vi "PathPlanner_Path_RePlan_Worker4.vi"(0 "JoinAnchor":T1 {"Y" format="%14.3f"; "X" format="%14.3f"}, 4 "StartingPoseTranslation":T1 {"Y" format="%14.3f"; "X" format="%14.3f"}, 5 "in PathPlannerPath":T2 {"AllPoints"."HolonomicRotation"."SIN" format="%13.4f"; "AllPoints"."HolonomicRotation"."COS" format="%13.4f"; "AllPoints"."HolonomicRotation"."VALUE" format="%13.4f"; "AllPoints"."Position"."Y" format="%14.3f"; "AllPoints"."Position"."X" format="%14.3f"; "GoalEndState"."Rotation"."SIN" format="%13.4f"; "GoalEndState"."Rotation"."COS" format="%13.4f"; "GoalEndState"."Rotation"."VALUE" format="%13.4f"; "RotationTargets"."target"."SIN" format="%13.4f"; "RotationTargets"."target"."COS" format="%13.4f"; "RotationTargets"."target"."VALUE" format="%13.4f"; "PreviewStartingRotation"."SIN" format="%13.4f"; "PreviewStartingRotation"."COS" format="%13.4f"; "PreviewStartingRotation"."VALUE" format="%13.4f"; "BezierPoints"."Y" format="%14.3f"; "BezierPoints"."X" format="%14.3f"}, 6 "robotNextCtrl":T1 {"Y" format="%14.3f"; "X" format="%14.3f"}, 7 "NumPtsMinusOne":i32, 9 "robotNextCtrl_NULL":bool, 10 "JoinPrevCtrl":T1 {"Y" format="%14.3f"; "X" format="%14.3f"}) -> (2 "Error":bool, 3 "Replanned Path":T2 {"AllPoints"."HolonomicRotation"."SIN" format="%13.4f"; "AllPoints"."HolonomicRotation"."COS" format="%13.4f"; "AllPoints"."HolonomicRotation"."VALUE" format="%13.4f"; "AllPoints"."Position"."Y" format="%14.3f"; "AllPoints"."Position"."X" format="%14.3f"; "GoalEndState"."Rotation"."SIN" format="%13.4f"; "GoalEndState"."Rotation"."COS" format="%13.4f"; "GoalEndState"."Rotation"."VALUE" format="%13.4f"; "RotationTargets"."target"."SIN" format="%13.4f"; "RotationTargets"."target"."COS" format="%13.4f"; "RotationTargets"."target"."VALUE" format="%13.4f"; "PreviewStartingRotation"."SIN" format="%13.4f"; "PreviewStartingRotation"."COS" format="%13.4f"; "PreviewStartingRotation"."VALUE" format="%13.4f"; "BezierPoints"."Y" format="%14.3f"; "BezierPoints"."X" format="%14.3f"})   [LabVIEW 2019, in "PathPlanner24.lvlib"]
doc: "Replan path worker 4\n\nInternal routine. Not for end user use."
uses:
  PathPlanner24.lvlib
  <vilib>/Rock Robotics/WPI/ThirdParty/JAS_Junk/TrajLib/Trajectory_Library.lvlib
  <vilib>/Rock Robotics/WPI/ThirdParty/JAS_Junk/TrajLib/TypeDef/ROTATION2D.ctl
  TypeDef/PathPlannerRotationTarget.ctl
  TypeDef/PathPlannerPathConstraints.ctl
  TypeDef/PathPlannerConstraintsZone.ctl
  ENum/PathPlanner_CommandUtilType_ENUM.ctl
  TypeDef/PathPlannerCommandUtil.ctl
  TypeDef/PathPlannerEventMarker.ctl
  <vilib>/Rock Robotics/WPI/ThirdParty/JAS_Junk/TrajLib/TypeDef/TRANSLATION2D.ctl
  TypeDef/PathPlannerGoalEndState.ctl
  TypeDef/PathPlannerPathPoint.ctl
  TypeDef/PathPlannerPath.ctl
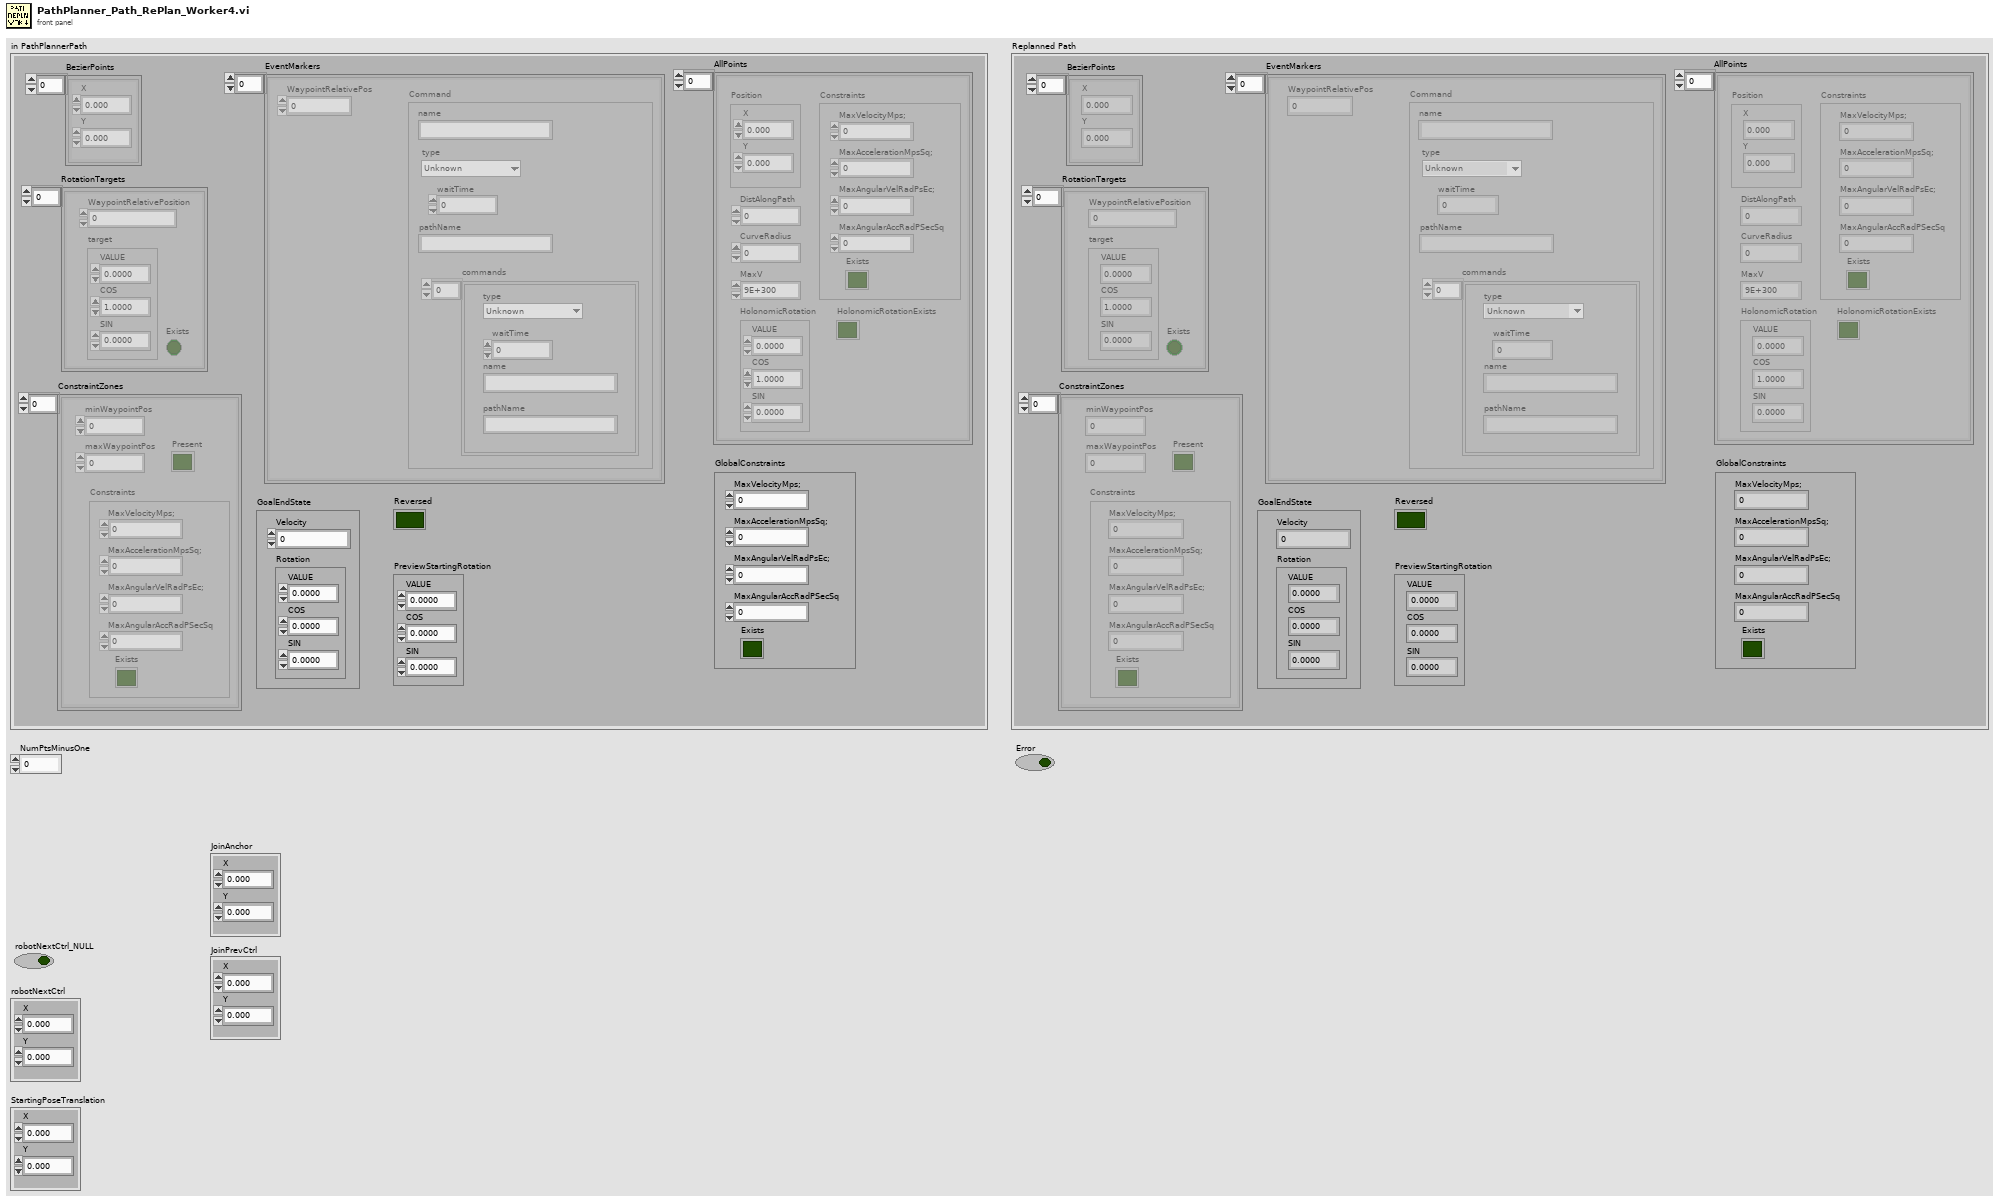
[diagram p1: front panel]
types:
  T1 = typedef "Trajectory_Library.lvlib/TRANSLATION2D.ctl" = cluster{"X":dbl, "Y":dbl}
  T2 = typedef "PathPlanner24.lvlib/PathPlannerPath.ctl" = cluster{"BezierPoints":T1[], "PreviewStartingRotation":T3, "Reversed":bool, "RotationTargets":T4[], "ConstraintZones":T5[], "EventMarkers":T7[], "GlobalConstraints":T6, "GoalEndState":T10, "AllPoints":T11[]}
  T3 = typedef "Trajectory_Library.lvlib/ROTATION2D.ctl" = cluster{"VALUE":dbl, "COS":dbl, "SIN":dbl}
  T4 = typedef "PathPlanner24.lvlib/PathPlannerRotationTarget.ctl" = cluster{"target":T3, "WaypointRelativePosition":dbl, "Exists":bool}
  T5 = typedef "PathPlanner24.lvlib/PathPlannerConstraintsZone.ctl" = cluster{"minWaypointPos":dbl, "maxWaypointPos":dbl, "Constraints":T6, "Present":bool}
  T6 = typedef "PathPlanner24.lvlib/PathPlannerPathConstraints.ctl" = cluster{"MaxVelocityMps;":dbl, "MaxAccelerationMpsSq;":dbl, "MaxAngularVelRadPsEc;":dbl, "MaxAngularAccRadPSecSq":dbl, "Exists":bool}
  T7 = typedef "PathPlanner24.lvlib/PathPlannerEventMarker.ctl" = cluster{"WaypointRelativePos":dbl, "Command":T8}
  T8 = typedef "PathPlanner24.lvlib/PathPlannerCommandUtil.ctl" = cluster{"waitTime":dbl, "name":string, "pathName":string, "commands":cluster{"type":T9, "waitTime":dbl, "name":string, "pathName":string}[], "type":T9}
  T9 = typedef "PathPlanner24.lvlib/PathPlanner_CommandUtilType_ENUM.ctl" = enum16{"Unknown", "Wait", "Named", "Path", "Sequential", "Parallel", "Race", "Deadline"}
  T10 = typedef "PathPlanner24.lvlib/PathPlannerGoalEndState.ctl" = cluster{"Velocity":dbl, "Rotation":T3}
  T11 = typedef "PathPlanner24.lvlib/PathPlannerPathPoint.ctl" = cluster{"Position":T1, "HolonomicRotation":T3, "DistAlongPath":dbl, "CurveRadius":dbl, "MaxV":dbl, "Constraints":T6, "HolonomicRotationExists":bool}
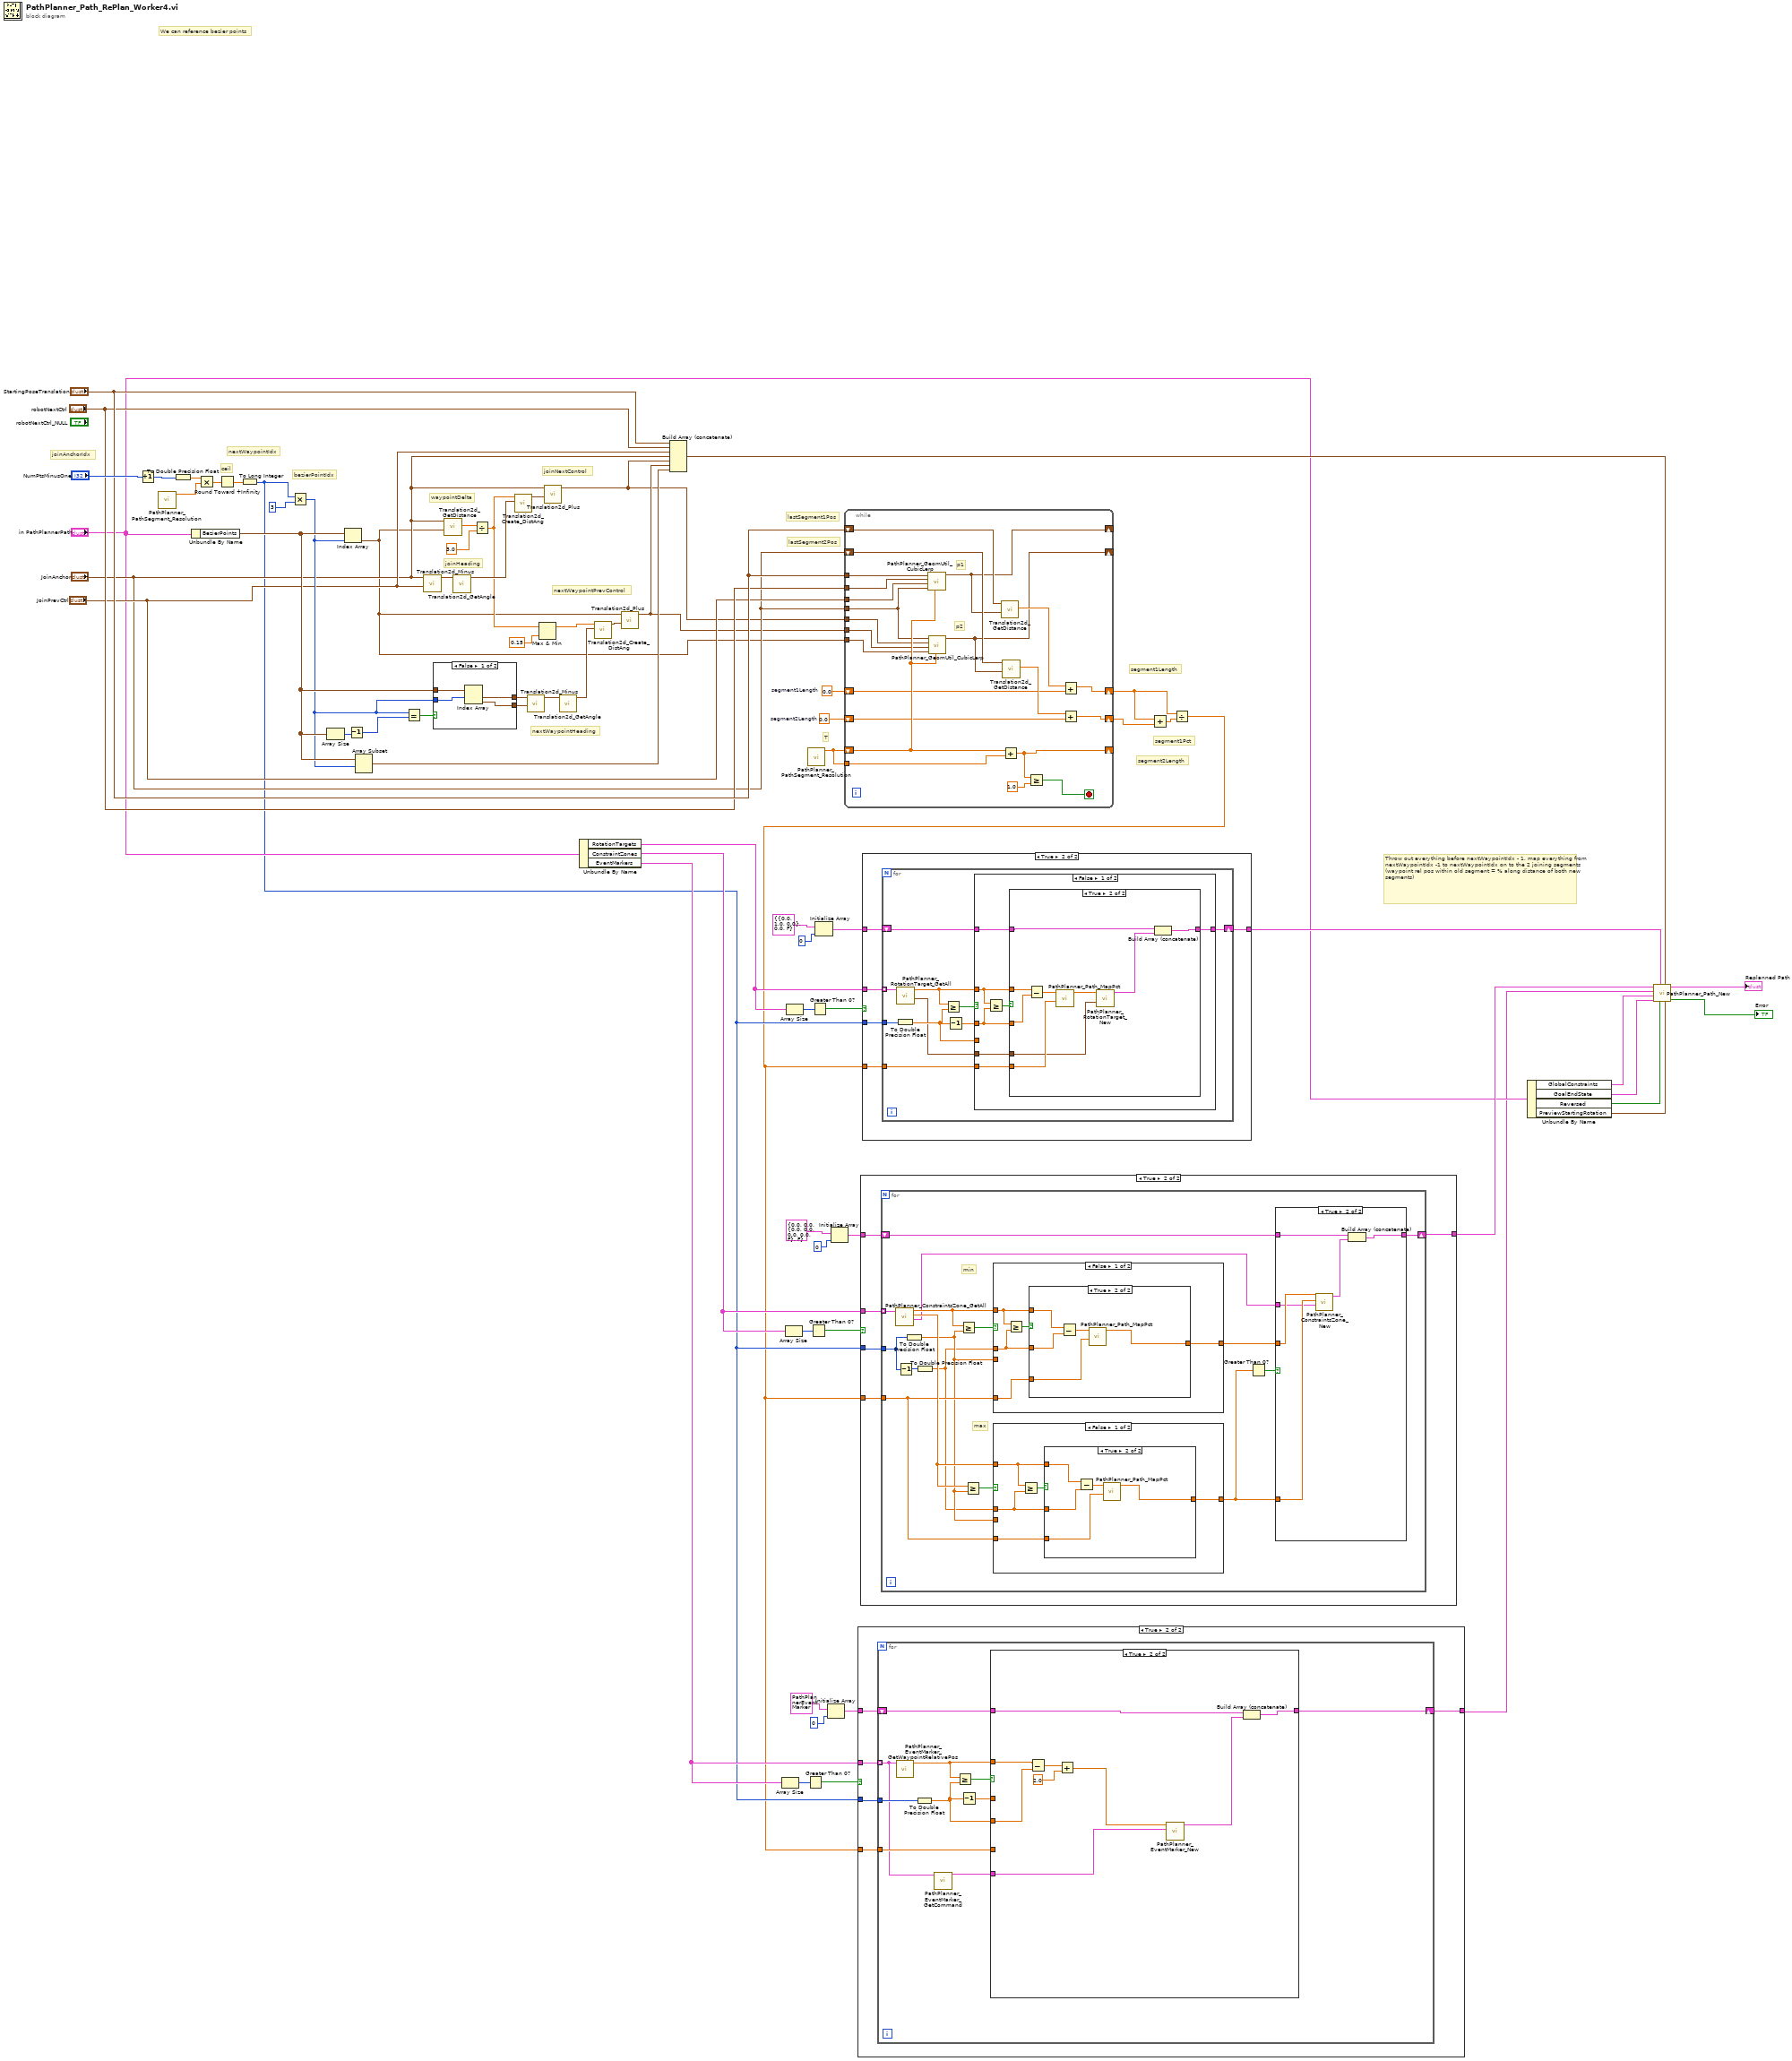
[diagram p0: block diagram]
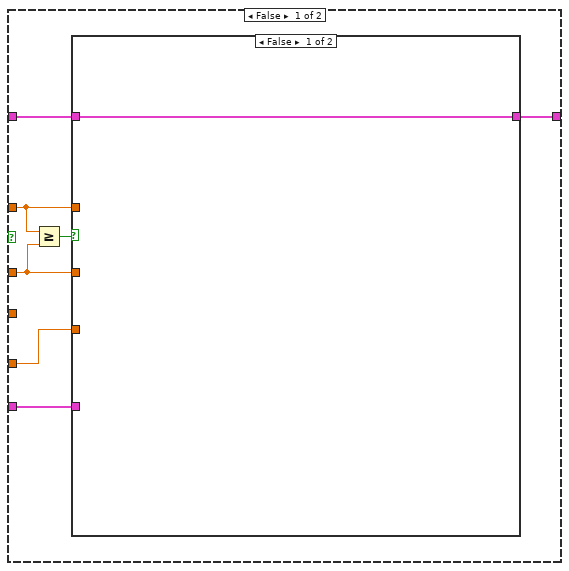
[diagram p3: hidden frame]
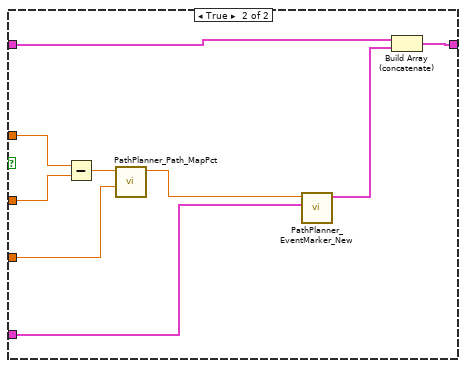
[diagram p4: hidden frame]
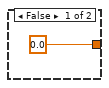
[diagram p7: hidden frame]
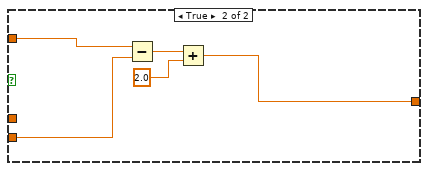
[diagram p8: hidden frame]
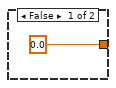
[diagram p9: hidden frame]
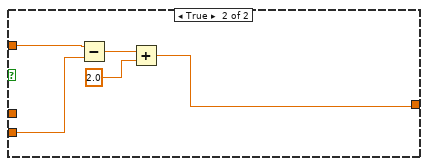
[diagram p10: hidden frame]
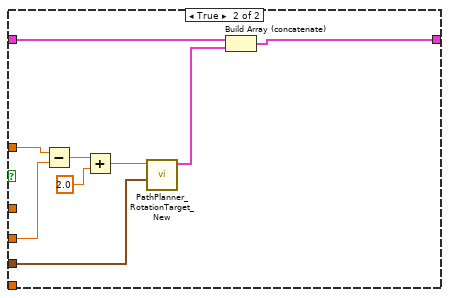
[diagram p13: hidden frame]
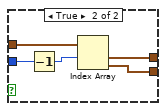
[diagram p14: hidden frame]
diagram:
  w43 = 0.0  # segment2Length
  w44 = 0.0  # segment1Length
  # "Throw out everything before nextWaypointIdx - 1, map everything from nextWaypointIdx -1 to nextWaypointIdx on to the 2 joining segments (waypoint rel pos within old segment = % along distance of both new segments)"
  # "segment2Length"
  # "segment1Length"
  # "segment1Pct"
  # "T"
  # "lastSegment2Pos"
  # "lastSegment1Pos"
  # "nextWaypointPrevControl"
  # "nextWaypointHeading"
  # "joinNextControl"
  # "joinHeading"
  # "waypointDelta"
  # "bezierPointIdx"
  # "nextWaypointIdx"
  # "ceil"
  # "We can reference bezier points"
  # "joinAnchorIdx"
  n1 = Increment(x="NumPtsMinusOne") -> (x+1=w69:i32)
  n2 = call "PathPlanner_PathSegment_Resolution.vi"() -> ("Resolution"=w67:dbl)  [unwired: 11 in]
  n3 = To Double Precision Float(number=w69) -> (double precision float=w68:dbl)
  n4 = Unbundle By Name("in PathPlannerPath") -> ("BezierPoints"=w47:T1[])
  n5 = Multiply(x=w68, y=w67) -> (x*y=w66:dbl)
  n6 = Round Toward +Infinity(x=w66) -> (ceil(x): smallest int >= x=w65:dbl)
  n7 = To Long Integer(number=w65) -> (32bit integer=w3:i32)
  n8 = Multiply(x=w3, y=3) -> (x*y=w46:i32)
  n9 = Array Size(array=w47) -> (size(s)=w57:i32)
  n10 = Index Array(array=w47, index=w46) -> (element=w35:T1)
  n11 = Decrement(x=w57) -> (x-1=w56:i32)
  n12 = Array Subset(array=w47, index=w46) -> (w45:T1[])  [unwired: 1 in]
  n13 = Equal?(x=w46, y=w56) -> (x = y?=w58:bool)
  n14 = call <vilib>:"Translation2d_Minus.vi"("other Translation"="JoinPrevCtrl", "In Translation"="JoinAnchor") -> ("Out Translation"=w63:T1)  [unwired: 9 in]
  n15 = case shown="False" w58 {
    tunnel: w46 -> [w73 w78]
    tunnel: w47 -> [w74 w77]
    tunnel: [w71 w76] -> w54
    tunnel: [w72 w75] -> w53
    frame False {
      n16 = Index Array(array=w74, index #1=w73) -> (element #1=w72:T1, element #2=w71:T1)  [unwired: 1 in]
    }
    frame True {
      n17 = Decrement(x=w78) -> (x-1=w79:i32)
      n18 = Index Array(array=w77, index #1=w79) -> (element #1=w75:T1, element #2=w76:T1)  [unwired: 1 in]
    }
  }
  n19 = call <vilib>:"Translation2d_GetDistance.vi"("other Translation"=w35, "In Translation"="JoinAnchor") -> ("Distance"=w60:dbl)  [unwired: 9 in]
  n20 = call <vilib>:"Translation2d_GetAngle.vi"("In Translation"=w63) -> ("Angle_Rotation2d"=w61:T3)  [unwired: 10 in]
  n21 = Divide(x=w60, y=3.0) -> (x/y=w52:dbl)
  n22 = call <vilib>:"Translation2d_Create_DistAng.vi"("Angle"=w61, "Dist"=w52) -> ("TRANSLATION"=w62:T1)  [unwired: 9 in]
  n23 = call <vilib>:"Translation2d_Minus.vi"("other Translation"=w54, "In Translation"=w53) -> ("Out Translation"=w55:T1)  [unwired: 9 in]
  n24 = Max & Min(x=w52, y=0.15 ("x")) -> (max(x,y)=w49:dbl)  [unwired: 1 out]
  n25 = call <vilib>:"Translation2d_Plus.vi"("other Translation"=w62, "In Translation"="JoinAnchor") -> ("Out Translation"=w36:T1)  [unwired: 9 in]
  n26 = call <vilib>:"Translation2d_GetAngle.vi"("In Translation"=w55) -> ("Angle_Rotation2d"=w50:T3)  [unwired: 10 in]
  n27 = Unbundle By Name("in PathPlannerPath") -> ("RotationTargets"=w26:T4[], "ConstraintZones"=w20:T5[], "EventMarkers"=w4:T7[])
  n28 = call <vilib>:"Translation2d_Create_DistAng.vi"("Angle"=w50, "Dist"=w49) -> ("TRANSLATION"=w48:T1)  [unwired: 9 in]
  n29 = call <vilib>:"Translation2d_Plus.vi"("other Translation"=w48, "In Translation"=w35) -> ("Out Translation"=w37:T1)  [unwired: 9 in]
  n30 = Build Array (concatenate)("StartingPoseTranslation", "robotNextCtrl", "JoinPrevCtrl", "JoinAnchor", w36, w37, w45) -> (w19:T1[])
  n31 = Array Size(array=w4) -> (size(s)=w6:i32)
  n32 = Array Size(array=w20) -> (size(s)=w22:i32)
  n33 = Array Size(array=w26) -> (size(s)=w28:i32)
  n34 = Greater Than 0?(x=w6) -> (x > 0?=w5:bool)
  n35 = call "PathPlanner_PathSegment_Resolution.vi"() -> ("Resolution"=w42:dbl)  [unwired: 11 in]
  n36 = Greater Than 0?(x=w22) -> (x > 0?=w21:bool)
  n37 = Greater Than 0?(x=w28) -> (x > 0?=w27:bool)
  n38 = Initialize Array(T4 {"target"={"VALUE"=0.0, "COS"=1.0, "SIN"=0.0}, "WaypointRelativePosition"=0.0, "Exists"=FALSE} ("RotationTarget"), 0 ("dimension size")) -> (w29:T4[])
  n39 = Initialize Array(T7 {"WaypointRelativePos"=0.0, "Command"={"waitTime"=0.0, "name"="", "pathName"="", "commands"=[], "type"=enum."Unknown"}} ("EventMarker"), 0 ("dimension size")) -> (w7:T7[])
  n40 = Initialize Array(T5 {"minWaypointPos"=0.0, "maxWaypointPos"=0.0, "Constraints"={"MaxVelocityMps;"=0.0, "MaxAccelerationMpsSq;"=0.0, "MaxAngularVelRadPsEc;"=0.0, "MaxAngularAccRadPSecSq"=0.0, "Exists"=FALSE}, "Present"=FALSE} ("ConstraintsZone"), 0 ("dimension size")) -> (w23:T5[])
  n41 = while {
    shift-right: [w83] -> w32
    shift-left: w44 -> [w85]
    shift-right: [w81] -> _
    shift-left: "StartingPoseTranslation" -> [w89]
    shift-right: [w82] -> w34
    shift-left: w43 -> [w84]
    shift-right: [w80] -> _
    shift-left: "JoinAnchor" -> [w88]
    shift-right: [w100] -> _
    shift-left: w42 -> [w94]
    tunnel: w42 -> [w101]
    tunnel: "StartingPoseTranslation" -> [w97]
    tunnel: "robotNextCtrl" -> [w96]
    tunnel: "JoinPrevCtrl" -> [w95]
    tunnel: "JoinAnchor" -> [w93]
    tunnel: w37 -> [w91]
    tunnel: w36 -> [w92]
    tunnel: w35 -> [w90]
    stop <- w98 stop-if-true
    # "p2"
    # "p1"
    n42 = call "PathPlanner_GeomUtil_CubicLerp.vi"("T"=w94, "D"=w93, "C"=w95, "B"=w96, "A"=w97) -> ("Lerp"=w81:T1)  [unwired: 6 in]
    n43 = call "PathPlanner_GeomUtil_CubicLerp.vi"("T"=w94, "D"=w90, "C"=w91, "B"=w92, "A"=w93) -> ("Lerp"=w80:T1)  [unwired: 6 in]
    n44 = call <vilib>:"Translation2d_GetDistance.vi"("other Translation"=w81, "In Translation"=w89) -> ("Distance"=w87:dbl)  [unwired: 9 in]
    n45 = Add(x=w94, y=w101) -> (x+y=w100:dbl)
    n46 = call <vilib>:"Translation2d_GetDistance.vi"("other Translation"=w80, "In Translation"=w88) -> ("Distance"=w86:dbl)  [unwired: 9 in]
    n47 = Greater Or Equal?(x=w100, y=1.0) -> (x >= y?=w98:bool)
    n48 = Add(x=w87, y=w85) -> (x+y=w83:dbl)
    n49 = Add(x=w86, y=w84) -> (x+y=w82:dbl)
  }
  n50 = Add(x=w32, y=w34) -> (x+y=w33:dbl)
  n51 = Divide(x=w32, y=w33) -> (x/y=w2:dbl)
  n52 = case shown="True" w5 {
    tunnel: w4 -> [_ w107]
    tunnel: w7 -> [w102 w106]
    tunnel: [w102 w105] -> w1
    tunnel: w3 -> [_ w104]
    tunnel: w2 -> [_ w103]
    frame False {
    }
    frame True {
      n53 = for {
        tunnel: w107 -> [w108] mode=indexing
        shift-right: [w110] -> w105
        shift-left: w106 -> [w111]
        tunnel: w104 -> [w114]
        tunnel: w103 -> [w116]
        n54 = call "PathPlanner_EventMarker_GetWaypointRelativePos.vi"("in EventMarker"=w108) -> ("WaypointRelativePos"=w115:dbl)  [unwired: 10 in]
        n55 = To Double Precision Float(number=w114) -> (double precision float=w112:dbl)
        n56 = call "PathPlanner_EventMarker_GetCommand.vi"("in EventMarker"=w108) -> ("Command"=w109:T8)  [unwired: 10 in]
        n57 = Greater Or Equal?(x=w115, y=w112) -> (x >= y?=w117:bool)
        n58 = Decrement(x=w112) -> (x-1=w113:dbl)
        n59 = case shown="True" w117 {
          tunnel: w115 -> [w123 w143]
          tunnel: w112 -> [_ w142]
          tunnel: w116 -> [w122 _]
          tunnel: w113 -> [w118 _]
          tunnel: w111 -> [w121 w138]
          tunnel: [w120 w137] -> w110
          tunnel: w109 -> [w119 w139]
          frame False {
            n60 = Greater Or Equal?(x=w123, y=w118) -> (x >= y?=w124:bool)
            n61 = case shown="False" w124 {
              tunnel: w123 -> [_ w133]
              tunnel: w122 -> [_ w132]
              tunnel: w121 -> [w125 w130]
              tunnel: [w125 w129] -> w120
              tunnel: w119 -> [_ w128]
              tunnel: w118 -> [_ w127]
              frame False {
              }
              frame True {
                n62 = Subtract(x=w133, y=w127) -> (x-y=w134:dbl)
                n63 = call "PathPlanner_Path_MapPct.vi"("Seg1Pct"=w132, "Pct"=w134) -> ("MapPct"=w126:dbl)  [unwired: 9 in]
                n64 = call "PathPlanner_EventMarker_New.vi"("Command"=w128, "WaypointRelativePos"=w126) -> ("EventMarker"=w131:T7)  [unwired: 9 in]
                n65 = Build Array (concatenate)(w130, w131) -> (w129:T7[])
              }
            }
          }
          frame True {
            n66 = Subtract(x=w143, y=w142) -> (x-y=w141:dbl)
            n67 = Add(x=w141, y=2.0) -> (x+y=w135:dbl)
            n68 = call "PathPlanner_EventMarker_New.vi"("Command"=w139, "WaypointRelativePos"=w135) -> ("EventMarker"=w136:T7)  [unwired: 9 in]
            n69 = Build Array (concatenate)(w138, w136) -> (w137:T7[])
          }
        }
      }
    }
  }
  n70 = case shown="True" w21 {
    tunnel: w20 -> [_ w149]
    tunnel: w23 -> [w144 w148]
    tunnel: [w144 w147] -> w17
    tunnel: w3 -> [_ w146]
    tunnel: w2 -> [_ w145]
    frame False {
    }
    frame True {
      n71 = for {
        tunnel: w149 -> [w165] mode=indexing
        shift-right: [w154] -> w147
        shift-left: w148 -> [w155]
        tunnel: w146 -> [w153]
        tunnel: w145 -> [w160]
        # "max"
        # "min"
        n72 = call "PathPlanner_ConstraintsZone_GetAll.vi"("ConstraintsZone"=w165) -> ("Constraints"=w156:T6, "maxWaypointPos"=w161:dbl, "minWaypointPos"=w162:dbl)  [unwired: 8 in]
        n73 = Decrement(x=w153) -> (x-1=w151:i32)
        n74 = To Double Precision Float(number=w153) -> (double precision float=w152:dbl)
        n75 = To Double Precision Float(number=w151) -> (double precision float=w150:dbl)
        n76 = Greater Or Equal?(x=w162, y=w152) -> (x >= y?=w164:bool)
        n77 = Greater Or Equal?(x=w161, y=w152) -> (x >= y?=w163:bool)
        n78 = case shown="False" w164 {
          tunnel: w162 -> [w191 w204]
          tunnel: w150 -> [w190 _]
          tunnel: [w192 w200] -> w158
          tunnel: w152 -> [_ w203]
          tunnel: w160 -> [w189 _]
          frame False {
            n79 = Greater Or Equal?(x=w191, y=w190) -> (x >= y?=w193:bool)
            n80 = case shown="True" w193 {
              tunnel: [0.0 w196] -> w192
              tunnel: w191 -> [_ w198]
              tunnel: w190 -> [_ w195]
              tunnel: w189 -> [_ w197]
              frame False {
              }
              frame True {
                n81 = Subtract(x=w198, y=w195) -> (x-y=w199:dbl)
                n82 = call "PathPlanner_Path_MapPct.vi"("Seg1Pct"=w197, "Pct"=w199) -> ("MapPct"=w196:dbl)  [unwired: 9 in]
              }
            }
          }
          frame True {
            n83 = Subtract(x=w204, y=w203) -> (x-y=w202:dbl)
            n84 = Add(x=w202, y=2.0) -> (x+y=w200:dbl)
          }
        }
        n85 = case shown="False" w163 {
          tunnel: w161 -> [w175 w186]
          tunnel: w150 -> [w174 _]
          tunnel: [w176 w184] -> w157
          tunnel: w152 -> [_ w185]
          tunnel: w160 -> [w173 _]
          frame False {
            n86 = Greater Or Equal?(x=w175, y=w174) -> (x >= y?=w177:bool)
            n87 = case shown="True" w177 {
              tunnel: [0.0 w180] -> w176
              tunnel: w175 -> [_ w183]
              tunnel: w174 -> [_ w179]
              tunnel: w173 -> [_ w181]
              frame False {
              }
              frame True {
                n88 = Subtract(x=w183, y=w179) -> (x-y=w182:dbl)
                n89 = call "PathPlanner_Path_MapPct.vi"("Seg1Pct"=w181, "Pct"=w182) -> ("MapPct"=w180:dbl)  [unwired: 9 in]
              }
            }
          }
          frame True {
            n90 = Subtract(x=w186, y=w185) -> (x-y=w188:dbl)
            n91 = Add(x=w188, y=2.0) -> (x+y=w184:dbl)
          }
        }
        n92 = Greater Than 0?(x=w157) -> (x > 0?=w159:bool)
        n93 = case shown="True" w159 {
          tunnel: w158 -> [_ w172]
          tunnel: w157 -> [_ w171]
          tunnel: w156 -> [_ w170]
          tunnel: w155 -> [w166 w169]
          tunnel: [w166 w167] -> w154
          frame False {
          }
          frame True {
            n94 = call "PathPlanner_ConstraintsZone_New.vi"("Constraints"=w170, "maxWaypointPos"=w171, "minWaypointPos"=w172) -> ("ConstraintsZone"=w168:T5)  [unwired: 8 in]
            n95 = Build Array (concatenate)(w169, w168) -> (w167:T5[])
          }
        }
      }
    }
  }
  n96 = case shown="True" w27 {
    tunnel: w26 -> [_ w210]
    tunnel: w29 -> [w205 w209]
    tunnel: [w205 w208] -> w18
    tunnel: w3 -> [_ w207]
    tunnel: w2 -> [_ w206]
    frame False {
    }
    frame True {
      n97 = for {
        tunnel: w210 -> [w220] mode=indexing
        shift-right: [w214] -> w208
        shift-left: w209 -> [w215]
        tunnel: w207 -> [w219]
        tunnel: w206 -> [w211]
        n98 = call "PathPlanner_RotationTarget_GetAll.vi"("RotationTarget"=w220) -> ("target"=w212:T3, "WaypointRelativePosition"=w217:dbl)  [unwired: 8 in, 1 out]
        n99 = To Double Precision Float(number=w219) -> (double precision float=w213:dbl)
        n100 = Greater Or Equal?(x=w217, y=w213) -> (x >= y?=w218:bool)
        n101 = Decrement(x=w213) -> (x-1=w216:dbl)
        n102 = case shown="False" w218 {
          tunnel: w217 -> [w223 w246]
          tunnel: w216 -> [w224 _]
          tunnel: w215 -> [w226 w240]
          tunnel: [w225 w238] -> w214
          tunnel: w213 -> [_ w245]
          tunnel: w212 -> [w221 w241]
          tunnel: w211 -> [w222 _]
          frame False {
            n103 = Greater Or Equal?(x=w223, y=w224) -> (x >= y?=w227:bool)
            n104 = case shown="True" w227 {
              tunnel: w226 -> [w228 w230]
              tunnel: [w228 w229] -> w225
              tunnel: w224 -> [_ w235]
              tunnel: w223 -> [_ w236]
              tunnel: w222 -> [_ w233]
              tunnel: w221 -> [_ w231]
              frame False {
              }
              frame True {
                n105 = Subtract(x=w236, y=w235) -> (x-y=w234:dbl)
                n106 = call "PathPlanner_Path_MapPct.vi"("Seg1Pct"=w233, "Pct"=w234) -> ("MapPct"=w232:dbl)  [unwired: 9 in]
                n107 = call "PathPlanner_RotationTarget_New.vi"("target"=w231, "WaypointRelativePosition"=w232) -> ("RotationTarget"=w237:T4)  [unwired: 9 in]
                n108 = Build Array (concatenate)(w230, w237) -> (w229:T4[])
              }
            }
          }
          frame True {
            n109 = Subtract(x=w246, y=w245) -> (x-y=w244:dbl)
            n110 = Add(x=w244, y=2.0) -> (x+y=w242:dbl)
            n111 = call "PathPlanner_RotationTarget_New.vi"("target"=w241, "WaypointRelativePosition"=w242) -> ("RotationTarget"=w239:T4)  [unwired: 9 in]
            n112 = Build Array (concatenate)(w240, w239) -> (w238:T4[])
          }
        }
      }
    }
  }
  n113 = Unbundle By Name("in PathPlannerPath") -> ("GlobalConstraints"=w15:T6, "GoalEndState"=w14:T10, "Reversed"=w13:bool, "PreviewStartingRotation"=w12:T3)
  n114 = call "PathPlanner_Path_New.vi"("PreviewStartingRotation"=w12, "BezierPoints"=w19, "Reversed"=w13, "HolonomicRotations"=w18, "GoalEndState"=w14, "GlobalConstraints"=w15, "EventMarkers"=w1, "ConstraintZones"=w17) -> ("Error"=→"Error":bool, "PathPlannerPath"=→"Replanned Path":T2)  [unwired: 2 in]
